vi "addSubWindow.vi"(8 "Error In":errorcluster, 9 "flags":T1 items=["Widget"=0, "Window"=1, "Dialog"=3, "Sheet"=5, "Drawer"=7, "Popup"=9, "Tool"=11, "ToolTip"=13, "SplashScreen"=15, "Desktop"=17, "SubWindow"=18, "ForeignWindow"=33, "CoverWindow"=65, "WindowType_Mask"=255, "MSWindowsFixedSizeDialogHint"=256, "MSWindowsOwnDC"=512, "BypassWindowManagerHint"=1024, "FramelessWindowHint"=2048, "WindowTitleHint"=4096, "WindowSystemMenuHint"=8192, "WindowMinimizeButtonHint"=16384, "WindowMaximizeButtonHint"=32768, "WindowMinMaxButtonsHint"=49152, "WindowContextHelpButtonHint"=65536, "WindowShadeButtonHint"=131072, "WindowStaysOnTopHint"=262144, "WindowTransparentForInput"=524288, "WindowOverridesSystemGestures"=1048576, "WindowDoesNotAcceptFocus"=2097152, "CustomizeWindowHint"=33554432, "WindowStaysOnBottomHint"=67108864, "WindowCloseButtonHint"=134217728, "MacWindowToolBarButtonHint"=268435456, "BypassGraphicsProxyWidget"=536870912, "NoDropShadowWindowHint"=1073741824, "WindowFullscreenButtonHint"=-2147483648], 10 "widget":refnum<class "QWidget.lvclass">, 11 "QMdiArea In":refnum<class "QMdiArea.lvclass">) -> (0 "Error Out":errorcluster, 2 "Value":refnum<class "QMdiSubWindow.lvclass">, 3 "QMdiArea Out":refnum<class "QMdiArea.lvclass">)   [LabVIEW 2014, in "QMdiArea.lvclass"]
doc: "LabVIEW-specific documentation is not yet available. See <b>http://doc.qt.io/qt-5/QMdiArea.html#addSubWindow</b>"
uses:
  QMdiArea.lvclass
  QMdiSubWindow/QMdiSubWindow.lvclass
  QWidget/QWidget.lvclass
  LQ Core/Qt/WindowType.ctl
  LQ Core/LQIdentity/LQIdentity.lvclass/LQIdentity.ctl
  LQ Core/LQ Core.lvlib
  LQ Core/LQIdentity/LQIdentity.lvclass
  LQ Core/LQCoreEngine/LQCoreEngine.lvclass
  LQ Core/Qt/Qt.lvlib
panel:
  # "Copyright (c) 2016 Sze Howe Koh\n\nThis Source Code Form is subject to the terms of the Mozilla Public\nLicense, v. 2.0. If a copy of the MPL was not distributed with this\nfile, You can obtain one at http://mozilla.org/MPL/2.0/."
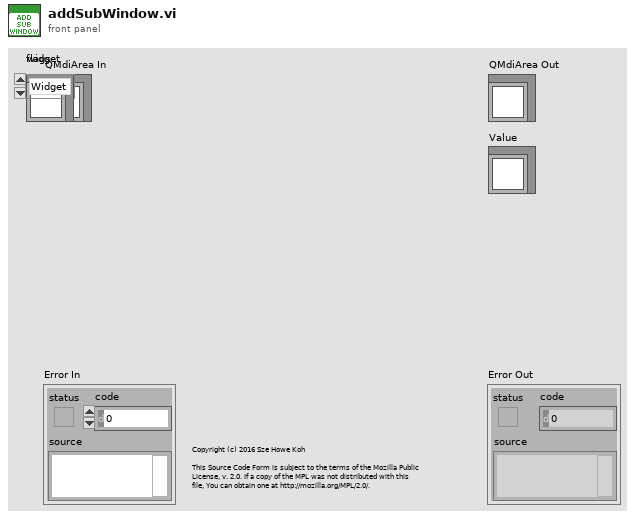
[diagram p1: front panel]
types:
  T1 = typedef "Qt.lvlib/WindowType.ctl" = i32
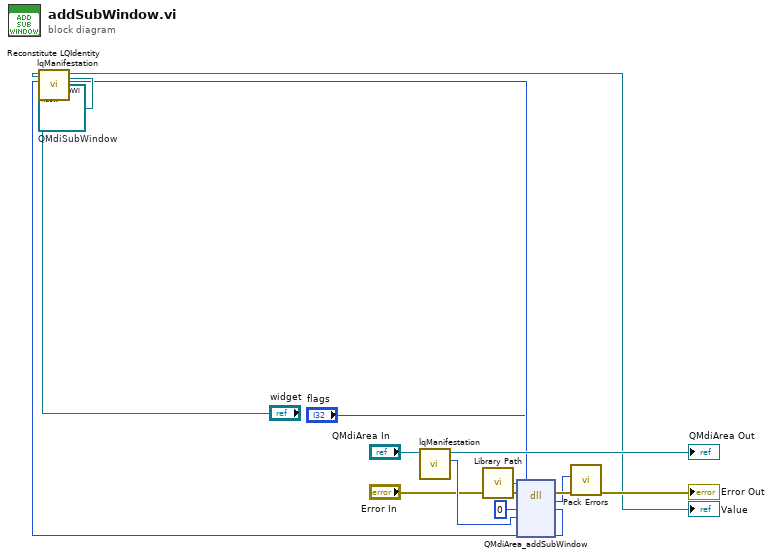
[diagram p0: block diagram]
diagram:
  w4 = refnum<class "QMdiSubWindow.lvclass"> refnum  # QMdiSubWindow
  n1 = call "lqManifestation.vi"("LQIdentity in"="widget") -> ("Manifestation"=w2:u64)  [unwired: 9 in, 1 out]
  n2 = call "lqManifestation.vi"("LQIdentity in"="QMdiArea In") -> ("Manifestation"=w11:u64, "LQIdentity out"=→"QMdiArea Out":refnum<class "QMdiArea.lvclass">)  [unwired: 9 in]
  n3 = call "Library Path.vi"() -> ("Library Path"=w12:path)
  n4 = dll-call lib="?" fn="QMdiArea_addSubWindow"(path in=w12, error in="Error In", "_retVal"=u64 0 ("retVal"), "_instance"=w11, "widget"=w2, "flags"="flags") -> (error out=w9:errorcluster, w7:i32, "_retVal"=w5:u64)  [unwired: 4 in, 1 out]
  n5 = call "Reconstitute LQIdentity.vi"("Manifestation"=w5, "LQIdentity Prototype"=w4) -> ("Reconstituted LQIdentity"=→"Value":refnum<class "QMdiSubWindow.lvclass">)  [unwired: 8 in, 1 out]
  n6 = call "Pack Errors.vi"("Error In"=w9, "Error Code"=w7) -> ("Error Out"=→"Error Out":errorcluster)  [unwired: 9 in]
